vi "Next_Action.vi"(4 "error in (no error)":errorcluster, 6 "Operations":T2(array[cluster]), 7 "queue in":refnum<queue>) -> (0 "error out":errorcluster, 2 "Operations Out":T1(array[cluster]), 3 "queue out":refnum<queue>)   [LabVIEW 2015]
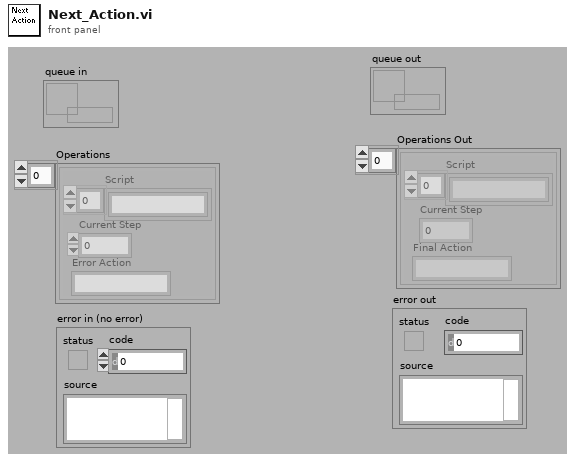
[diagram p1: front panel]
types:
  T1 = cluster{"Script":string[], "Final Action":string, "Current Step":i32}[]
  T2 = cluster{"Script":string[], "Error Action":string, "Current Step":i32}[]
  T3 = cluster{"Script":string[], "Error Action":string, "Current Step":i32}
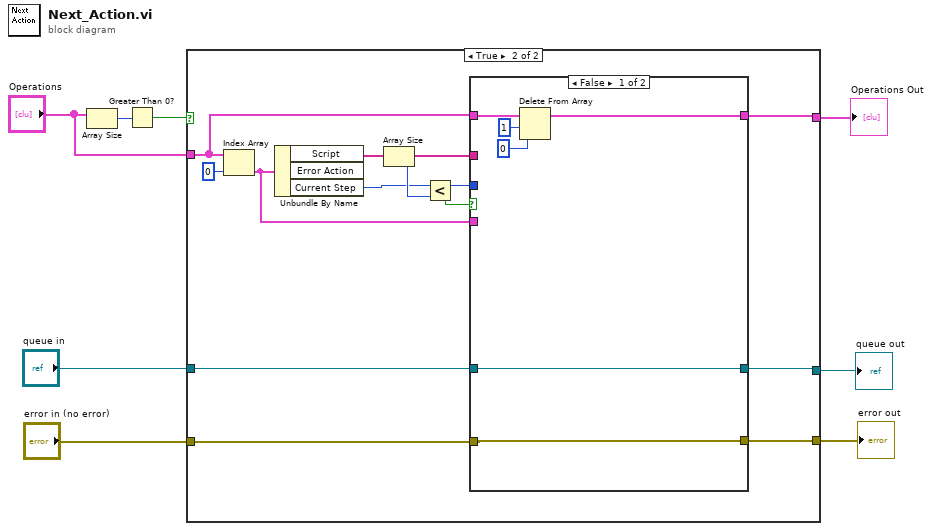
[diagram p0: block diagram]
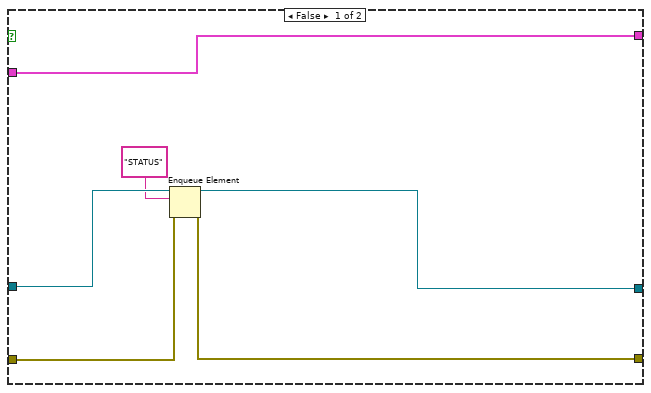
[diagram p2: hidden frame]
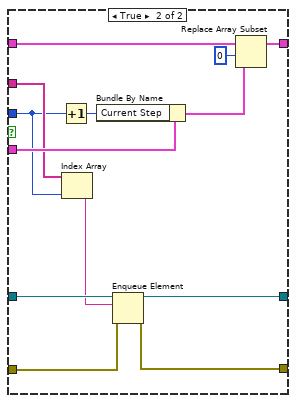
[diagram p3: hidden frame]
diagram:
  n1 = Array Size(array="Operations") -> (size(s)=w8:i32)
  n2 = Greater Than 0?(x=w8) -> (x > 0?=w7:bool)
  n3 = case shown="True" w7 {
    tunnel: "Operations" -> [w9 w25]
    tunnel: "queue in" -> [w14 w23]
    tunnel: [w13 w15] -> w4
    tunnel: "error in (no error)" -> [w12 w22]
    tunnel: [w11 w16] -> w2
    tunnel: [w9 w19] -> w1
    frame False {
      n4 = Enqueue Element(queue=w14, element="STATUS", error in (no error)=w12) -> (queue out=w13:refnum<queue>, error out=w11:errorcluster)  [unwired: 1 in, 1 out]
    }
    frame True {
      n5 = Index Array(array=w25, index=0) -> (element=w24:T3)
      n6 = Unbundle By Name(w24) -> ("Script"=w17:string[], "Current Step"=w20:i32)  [unwired: 1 out]
      n7 = Array Size(array=w17) -> (size(s)=w26:i32)
      n8 = Less?(x=w20, y=w26) -> (x < y?=w21:bool)
      n9 = case shown="False" w21 {
        tunnel: w25 -> [w32 w42]
        tunnel: w24 -> [_ w45]
        tunnel: w23 -> [w28 w37]
        tunnel: w22 -> [w27 w36]
        tunnel: w20 -> [_ w38]
        tunnel: [w31 w43] -> w19
        tunnel: w17 -> [_ w39]
        tunnel: [w27 w35] -> w16
        tunnel: [w28 w34] -> w15
        frame False {
          n10 = Delete From Array(array=w32, length=1, index=0) -> (array with subset deleted=w31:T2)  [unwired: 1 out]
        }
        frame True {
          n11 = Increment(x=w38) -> (x+1=w44:i32)
          n12 = Index Array(array=w39, index=w38) -> (element=w33:string)
          n13 = Bundle By Name(cluster=w45, "Current Step"=w44) -> (w40:T3)
          n14 = Enqueue Element(queue=w37, element=w33, error in (no error)=w36) -> (queue out=w34:refnum<queue>, error out=w35:errorcluster)  [unwired: 1 in, 1 out]
          n15 = Replace Array Subset(array=w42, new element=w40, index=0) -> (w43:T2)
        }
      }
    }
  }
  "queue out" <- w4
  "error out" <- w2
  "Operations Out" <- w1
